vi "matrix_multiply.vi"(1 "p":i32, 2 "C":sgl[](array[numeric]), 3 "n":i32, 4 "m":i32, 5 "B":sgl[](array[numeric]), 6 "A":sgl[](array[numeric])) -> (0 "C":sgl[](array[numeric]))   [LabVIEW 2020]
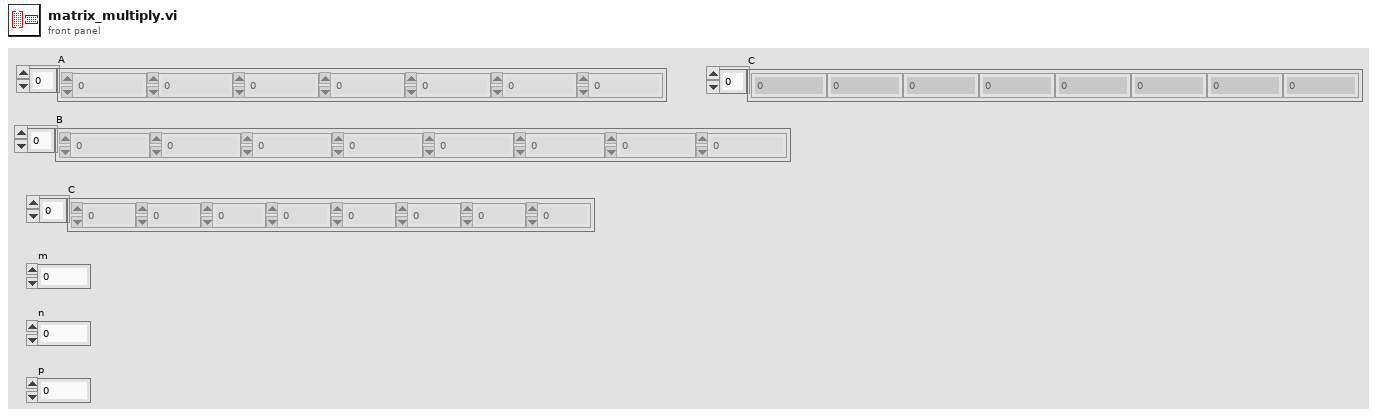
[diagram p1: front panel]
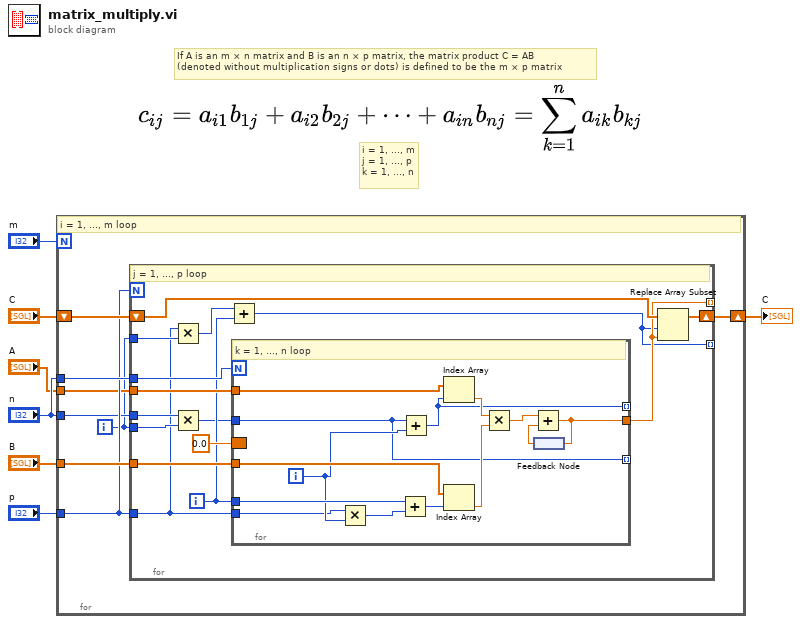
[diagram p0: block diagram]
diagram:
  # "If A is an m × n matrix and B is an n × p matrix, the matrix product C = AB \n(denoted without multiplication signs or dots) is defined to be the m × p matrix"
  # "i = 1, ..., m\nj = 1, ..., p\nk = 1, ..., n"
  n1 = for {
    N: "m" -> [_]
    tunnel: "B" -> [w15]
    tunnel: "n" -> [w14]
    tunnel: "p" -> [w11]
    tunnel: "A" -> [w10]
    tunnel: "n" -> [w9]
    shift-right: [w12] -> w3
    shift-left: "C" -> [w13]
    i -> [w8]
    # "i = 1, ..., m loop"
    n2 = for {
      N: w11 -> [_]
      tunnel: w10 -> [w30]
      tunnel: w15 -> [w29]
      tunnel: w14 -> [w23]
      tunnel: w11 -> [w16]
      tunnel: [w25] -> _ mode=indexing
      tunnel: [w24] -> _ mode=indexing
      shift-right: [w26] -> w12
      shift-left: w13 -> [w27]
      tunnel: w8 -> [w21]
      tunnel: w9 -> [w19]
      tunnel: w8 -> [w17]
      i -> [w22]
      # "j = 1, ..., p loop"
      n3 = Multiply(x=w16, y=w21) -> (x*y=w20:i32)
      n4 = Multiply(x=w19, y=w17) -> (x*y=w18:i32)
      n5 = Add(x=w20, y=w22) -> (x+y=w24:i32)
      n6 = for {
        N: w23 -> [_]
        tunnel: w30 -> [w44]
        tunnel: w18 -> [w31]
        tunnel: w29 -> [w43]
        tunnel: w22 -> [w37]
        tunnel: [w38] -> w25
        tunnel: w16 -> [w35]
        tunnel: [w32] -> _ mode=indexing
        border: sgl 0.0 -> [_]
        tunnel: [w31] -> _ mode=indexing
        i -> [w36]
        # "k = 1, ..., n loop"
        n7 = Multiply(x=w35, y=w36) -> (x*y=w34:i32)
        n8 = Add(x=w37, y=w34) -> (x+y=w33:i32)
        n9 = Add(x=w31, y=w36) -> (x+y=w32:i32)
        n10 = Index Array(array=w44, index=w32) -> (element=w42:sgl)
        n11 = Index Array(array=w43, index=w33) -> (element=w41:sgl)
        n12 = Multiply(x=w42, y=w41) -> (x*y=w40:sgl)
        n13 = feedback #1() -> (w39:sgl)
        n14 = Add(x=w40, y=w39) -> (x+y=w38:sgl)
        n15 = feedback-in #1(w38) -> ()
      }
      n16 = Replace Array Subset(array=w27, new element=w25, index=w24) -> (w26:sgl[])
    }
  }
  "C" <- w3
